vi "get-edges.vi"(8 "error in (no error)":errorcluster, 11 "Graph in":refnum<class "Graph.lvclass">) -> (0 "error out":errorcluster, 2 "edges":set{T1}(c389), 3 "Graph out":refnum<class "Graph.lvclass">)   [LabVIEW 2020, in "graph.lvlib" / "Graph.lvclass"]
uses:
  Graph.lvclass
  Graph.lvclass/Graph.ctl
  4cd1d20b-5177-45a0-93a9-486eb44cea57.vi
  8a808ed8-a4e0-45c0-bfd1-75403d0b1c0b.vi
  ID/ID.lvclass
  edge-definition-cluster.ctl
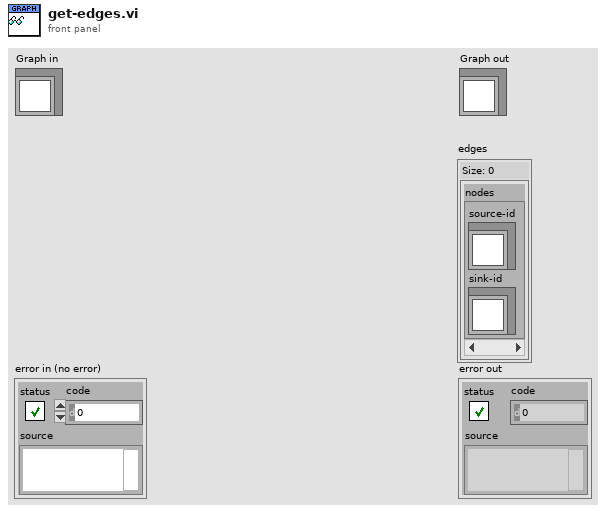
[diagram p1: front panel]
types:
  T1 = typedef "graph.lvlib/Graph.lvclass/edge-definition-cluster.ctl" = cluster{"source-id":refnum<class "ID.lvclass">, "sink-id":refnum<class "ID.lvclass">}
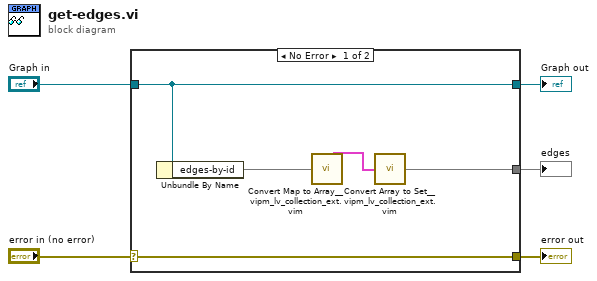
[diagram p0: block diagram]
diagram:
  n1 = case shown="No Error" "error in (no error)" {
    selector: "error in (no error)" -> [w10 w11]
    tunnel: [w10 w11] -> w4
    tunnel: [w9 w12] -> w2
    tunnel: "Graph in" -> [w9 w12]
    tunnel: [w6 _] -> w1
    frame No Error {
      n2 = Unbundle By Name(w9) -> ("edges-by-id"=w8:map{T1, refnum<class "Edge.lvclass">})
      n3 = call "Convert Map to Array__vipm_lv_collection_ext.vim"("map"=w8) -> ("keys"=w7:T1[])  [unwired: 12 in, 2 out]
      n4 = call "Convert Array to Set__vipm_lv_collection_ext.vim"("array"=w7) -> ("set"=w6:set{T1})  [unwired: 6 in]
    }
    frame Error {
    }
  }
  "error out" <- w4
  "Graph out" <- w2
  "edges" <- w1
